vi "Update Sender.vi"(10 "Debug Data.lvclass":refnum<class "Debug Data.lvclass">, 11 "Debug Log in":refnum<class "Debug Log.lvclass">) -> (2 "Debug Data out":refnum<class "Debug Data.lvclass">, 3 "Debug Log out":refnum<class "Debug Log.lvclass">)   [LabVIEW 2020, in "Debug Log.lvclass"]
uses:
  Debug Log.lvclass
  Debug Data/Debug Data.lvclass
  Debug Data/Debug Data.lvclass/Debug Data.ctl
  Debug Log.lvclass/Debug Log.ctl
  <vilib>/Utility/miscctls.llb/LVMapReplaceAction.ctl
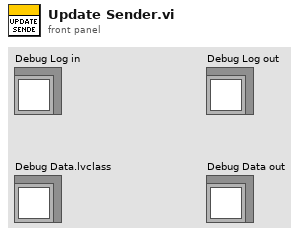
[diagram p1: front panel]
types:
  T1 = typedef "LVMapReplaceAction.ctl" = enum32{"Modify Entry only if found", "Add or Modify Entry", "Delete Entry"}
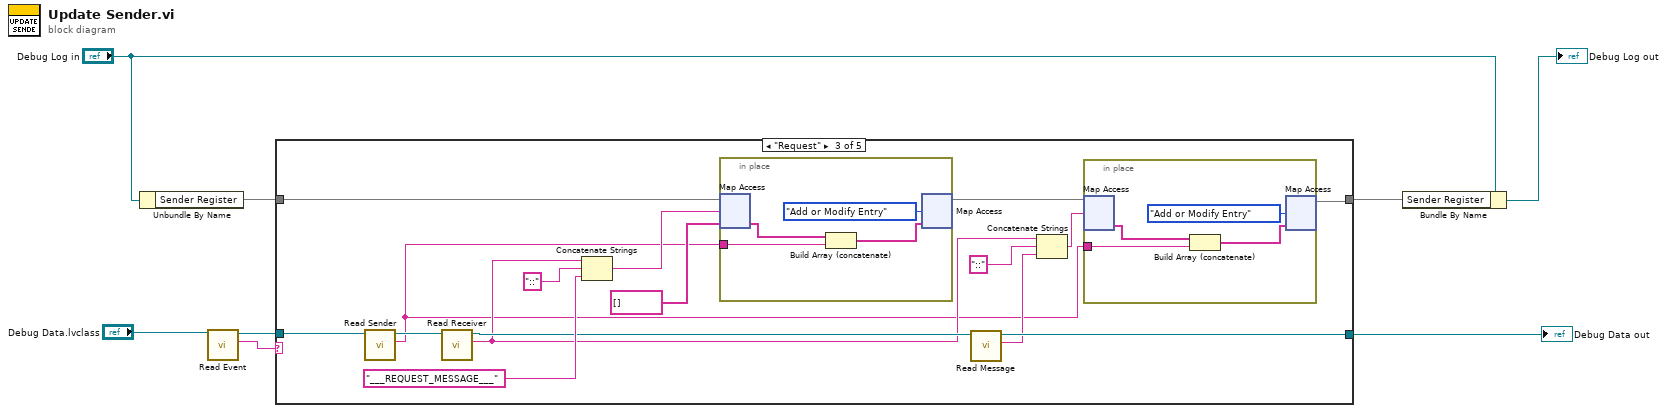
[diagram p0: block diagram]
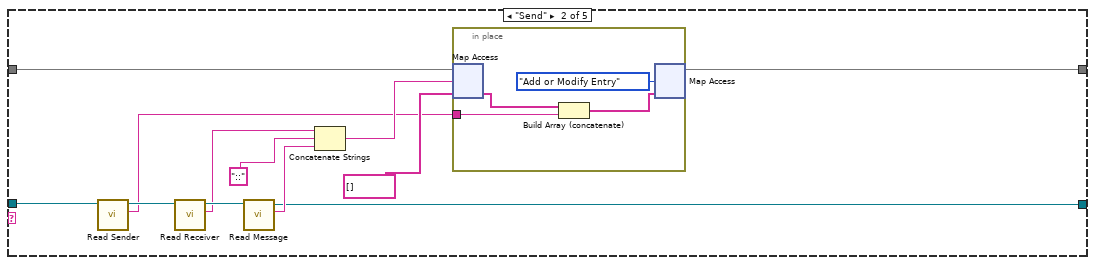
[diagram p3: hidden frame]
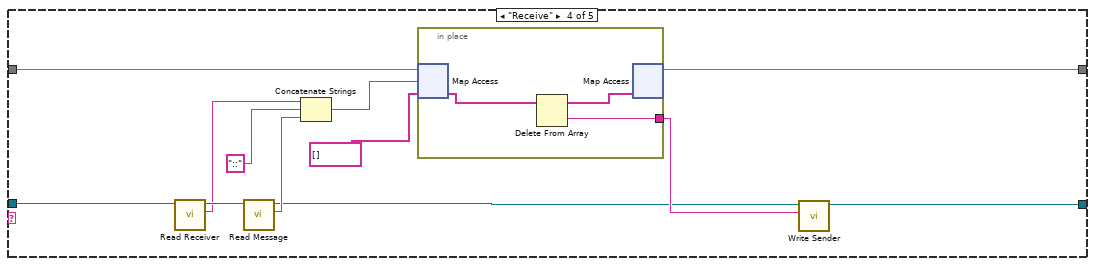
[diagram p4: hidden frame]
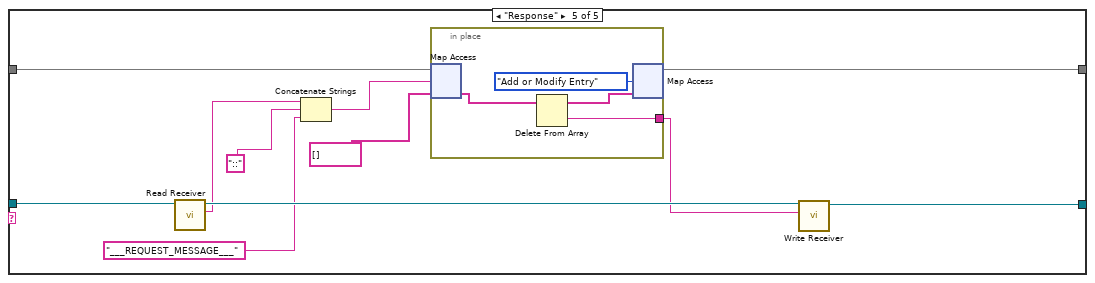
[diagram p5: hidden frame]
diagram:
  n1 = Unbundle By Name("Debug Log in") -> ("Sender Register"=w8:map{string, string[]})
  n2 = call "Read Event.vi"("Debug Data in"="Debug Data.lvclass") -> ("Event"=w4:string, "Debug Data out"=w3:refnum<class "Debug Data.lvclass">)  [unwired: 9 in]
  n3 = case shown="\"Request\"" w4 {
    tunnel: w3 -> [w9 w22 w42 w62 w76]
    tunnel: [w10 w13 w34 w55 w70] -> w6
    tunnel: w8 -> [w10 w12 w37 w54 w69]
    tunnel: [w9 w11 w32 w51 w67] -> w2
    frame Default {
    }
    frame "Send" {
      n4 = call "Read Sender.vi"("Debug Data In"=w22) -> ("Sender"=w14:string, "Debug Data Out"=w20:refnum<class "Debug Data.lvclass">)  [unwired: 9 in]
      n5 = call "Read Receiver.vi"("Debug Data In"=w20) -> ("Receiver"=w19:string, "Debug Data Out"=w21:refnum<class "Debug Data.lvclass">)  [unwired: 9 in]
      n6 = call "Read Message.vi"("Debug Data in"=w21) -> ("Message"=w18:string, "Debug Data out"=w11:refnum<class "Debug Data.lvclass">)  [unwired: 8 in, 1 out]
      n7 = Concatenate Strings(w19, "::" ("string"), w18) -> (w16:string)
      n8 = in-place {
        in-place-border: w14 -> [w24]
        n9 = in-place-map #1(w12, w16, string[] [] ("Sender")) -> (w25:string[])  [unwired: 1 out]
        n10 = Build Array (concatenate)(w25, w24) -> (w23:string[])
        n11 = in-place-map #1(w23, LVMapReplaceAction."Add or Modify Entry" ("action")) -> (w13:map{string, string[]})  [unwired: 2 out]
      }
    }
    frame "Request" {
      n12 = call "Read Sender.vi"("Debug Data In"=w42) -> ("Sender"=w27:string, "Debug Data Out"=w41:refnum<class "Debug Data.lvclass">)  [unwired: 9 in]
      n13 = call "Read Receiver.vi"("Debug Data In"=w41) -> ("Receiver"=w30:string, "Debug Data Out"=w33:refnum<class "Debug Data.lvclass">)  [unwired: 9 in]
      n14 = Concatenate Strings(w30, "::" ("string"), "___REQUEST_MESSAGE___" ("string")) -> (w39:string)
      n15 = in-place {
        in-place-border: w27 -> [w48]
        n16 = in-place-map #2(w37, w39, string[] [] ("Sender")) -> (w49:string[])  [unwired: 1 out]
        n17 = Build Array (concatenate)(w49, w48) -> (w47:string[])
        n18 = in-place-map #2(w47, LVMapReplaceAction."Add or Modify Entry" ("action")) -> (w35:map{string, string[]})  [unwired: 2 out]
      }
      n19 = call "Read Message.vi"("Debug Data in"=w33) -> ("Message"=w29:string, "Debug Data out"=w32:refnum<class "Debug Data.lvclass">)  [unwired: 8 in, 1 out]
      n20 = Concatenate Strings(w30, "::" ("string"), w29) -> (w28:string)
      n21 = in-place {
        in-place-border: w27 -> [w44]
        n22 = in-place-map #3(w35, w28) -> (w45:string[])  [unwired: 1 in, 1 out]
        n23 = Build Array (concatenate)(w45, w44) -> (w43:string[])
        n24 = in-place-map #3(w43, LVMapReplaceAction."Add or Modify Entry" ("action")) -> (w34:map{string, string[]})  [unwired: 2 out]
      }
    }
    frame "Receive" {
      n25 = call "Read Receiver.vi"("Debug Data In"=w62) -> ("Receiver"=w60:string, "Debug Data Out"=w61:refnum<class "Debug Data.lvclass">)  [unwired: 9 in]
      n26 = call "Read Message.vi"("Debug Data in"=w61) -> ("Message"=w59:string, "Debug Data out"=w52:refnum<class "Debug Data.lvclass">)  [unwired: 8 in, 1 out]
      n27 = Concatenate Strings(w60, "::" ("string"), w59) -> (w57:string)
      n28 = in-place {
        in-place-border: [w63] -> w53
        n29 = in-place-map #4(w54, w57, string[] [] ("Sender")) -> (w65:string[])  [unwired: 1 out]
        n30 = Delete From Array(array=w65) -> (deleted portion=w63:string, array with subset deleted=w64:string[])  [unwired: 2 in]
        n31 = in-place-map #4(w64) -> (w55:map{string, string[]})  [unwired: 1 in, 2 out]
      }
      n32 = call "Write Sender.vi"("Sender"=w53, "Debug Data In"=w52) -> ("Debug Data Out"=w51:refnum<class "Debug Data.lvclass">)  [unwired: 9 in]
    }
    frame "Response" {
      n33 = call "Read Receiver.vi"("Debug Data In"=w76) -> ("Receiver"=w74:string, "Debug Data Out"=w75:refnum<class "Debug Data.lvclass">)  [unwired: 9 in]
      n34 = Concatenate Strings(w74, "::" ("string"), "___REQUEST_MESSAGE___" ("string")) -> (w72:string)
      n35 = in-place {
        in-place-border: [w77] -> w68
        n36 = in-place-map #5(w69, w72, string[] [] ("Sender")) -> (w79:string[])  [unwired: 1 out]
        n37 = Delete From Array(array=w79) -> (deleted portion=w77:string, array with subset deleted=w78:string[])  [unwired: 2 in]
        n38 = in-place-map #5(w78, LVMapReplaceAction."Add or Modify Entry" ("action")) -> (w70:map{string, string[]})  [unwired: 2 out]
      }
      n39 = call "Write Receiver.vi"("Receiver"=w68, "Debug Data In"=w75) -> ("Debug Data Out"=w67:refnum<class "Debug Data.lvclass">)  [unwired: 9 in]
    }
  }
  "Debug Data out" <- w2
  n40 = Bundle By Name(cluster="Debug Log in", "Sender Register"=w6) -> (→"Debug Log out":refnum<class "Debug Log.lvclass">)
